vi "_EnumEditor_GetVI_Type.vi"(8 "error in (no error)":errorcluster, 11 "_EnumEditor in":refnum<class "_EnumEditor.lvclass">) -> (0 "error out":errorcluster, 2 "Control VI Type":T1(ring), 3 "_EnumEditor out":refnum<class "_EnumEditor.lvclass">)   [LabVIEW 2014, in "_EnumEditor.lvclass"]
uses:
  _EnumEditor.lvclass
  _EnumEditor.lvclass/_EnumEditor.ctl
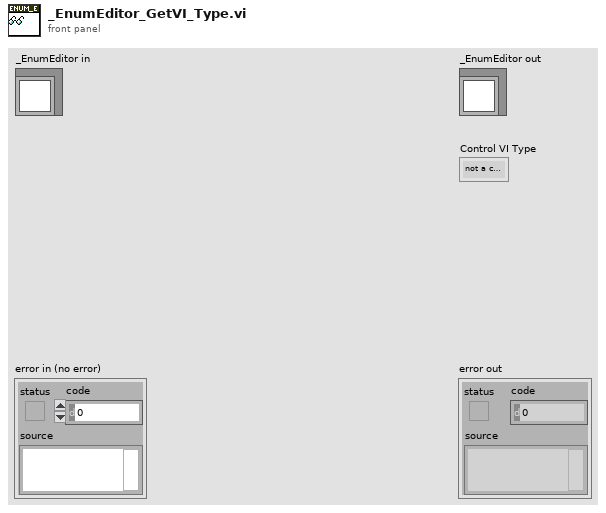
[diagram p1: front panel]
types:
  T1 = enum32{"not a control VI", "control", "typedef", "strict typedef"}
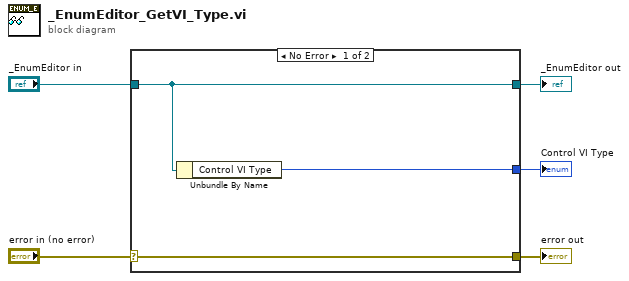
[diagram p0: block diagram]
diagram:
  n1 = case shown="No Error" "error in (no error)" {
    selector: "error in (no error)" -> [w8 w9]
    tunnel: [w8 w9] -> w4
    tunnel: [w7 w10] -> w2
    tunnel: "_EnumEditor in" -> [w7 w10]
    tunnel: [w6 _] -> w1
    frame No Error {
      n2 = Unbundle By Name(w7) -> ("Control VI Type"=w6:T1)
    }
    frame Error {
    }
  }
  "error out" <- w4
  "_EnumEditor out" <- w2
  "Control VI Type" <- w1
